vi "Cleanup.vi"(8 "error in (no error)":errorcluster, 11 "ByRef Mul in":refnum<class "ByRef Mul.lvclass">) -> (0 "error out":errorcluster)   [LabVIEW 2020, in "ByRef Mul.lvclass"]
uses:
  ByRef Mul.lvclass
  ByRef Base/ByRef Base.lvclass
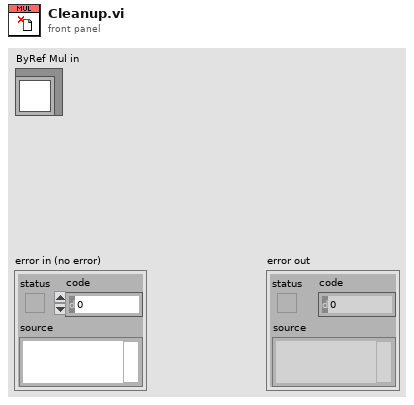
[diagram p1: front panel]
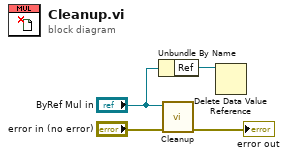
[diagram p0: block diagram]
diagram:
  n1 = Unbundle By Name("ByRef Mul in") -> ("Ref"=w1:refnum<data-value>)
  n2 = call-parent "Cleanup.vi"("error in (no error)"="error in (no error)", "ByRef Base in"="ByRef Mul in") -> ("error out"=→"error out":errorcluster)  [unwired: 9 in]
  n3 = Delete Data Value Reference(data value reference=w1) -> ()  [unwired: 1 in, 2 out]
